vi "Get Current Position Raw.vi"(8 "error in":errorcluster, 11 "Gantry in":refnum<class "Gantry.lvclass">) -> (0 "error out":errorcluster, 2 "Vec3d Class out":refnum<class "Vec3d.lvclass">, 3 "Gantry out":refnum<class "Gantry.lvclass">)   [LabVIEW 2026, in "Gantry.lvclass"]
uses:
  Gantry.lvclass
  Vec3d Class/Vec3d.lvclass
  Gantry.lvclass/Gantry.ctl
  <instrlib>/Aerotech Automation1/Status/TypeDefs/Axis Status Items Cluster.ctl
  <instrlib>/Aerotech Automation1/Status/TypeDefs/Axis Status Item.ctl
  <instrlib>/Aerotech Automation1/Status/Wrappers/Add Axis Status Item.vi
  <instrlib>/Aerotech Automation1/Status/Wrappers/Read Axis Status Item.vi
  <instrlib>/Aerotech Automation1/Status/Status.lvlib
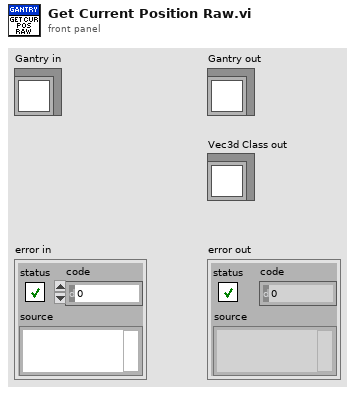
[diagram p1: front panel]
types:
  T1 = typedef "Virtual Modes.ctl" = enum16{"Nonvirtual", "Virtual"}
  T2 = typedef "ControllerDiagPacket.ctl" = cluster{"Number of Diag Packets":i32, "Axes":T3[], "error":errorcluster}
  T3 = typedef "AxisDiagPacket.ctl" = cluster{"Axis Name":string, "Analog Input 0":dbl, "Analog Input 1":dbl, "Axis Fault (num)":i32, "Axis Fault (str)":string, "Axis Fault (bits)":cluster{"AmplifierFault":bool, "AmplifierTemperatureFault":bool, "CcwEndOfTravelLimitFault":bool, "CcwSoftwareLimitFault":bool, "CommunicationLostFault":bool, "CwEndOfTravelLimitFault":bool, "CwSoftwareLimitFault":bool, "EmergencyStopFault":bool, "EncoderFault":bool, "ExternalFault":bool, "FeedbackScalingFault":bool, "GantryMisalignFault ":bool, "HallSensorFault":bool, "InPositionTimeoutFault":bool, "InternalFault":bool, "MarkerSearchFault":bool, "MaxVelocityCommandFault":bool, "MissedInterruptFault":bool, "MotorTemperatureFault":bool, "None":bool, "OverCurrentFault":bool, "PositionErrorFault":bool, "PositionFeedbackFault":bool, "PowerSupplyFault":bool, "ProbeInputFault":bool, "SafeZoneFault":bool, "VelocityErrorFault":bool, "VelocityFeedbackFault":bool, "VoltageClampFault":bool}, "Axis Status (num)":i32, "Axis Status (str)":string, "Axis Status (bits)":cluster{"BacklashActive":bool, "CalibrationEnabled1D":bool, "CalibrationEnabled2D":bool, "CommandValid":bool, "DriveAbortPending":bool, "DrivePending":bool, "Enabling":bool, "GainMappingEnabled":bool, "GantryAligned":bool, "GantryRealigning":bool, "Homed":bool, "Homing":bool, "IFOVEnabled":bool, "JogGenerating":bool, "Jogging":bool, "JoystickControl":bool, "MasterSlaveControl":bool, "MotionBlocked":bool, "MotionClamped":bool, "MoveDone":bool, "None":bool, "NotVirtual":bool, "Profiling":bool, "Stability0":bool, "Stability1":bool, "TrajectoryFiltering":bool, "WaitDone":bool}, "Current Command":sgl, "Current Error":sgl, "Current Feedback":sgl, "Digital Inputs":i32, "Digital Outputs":i32, "Drive Status":i32, "Drive Status (str)":string, "Drive Status (bits)":cluster{"AccelerationPhase":bool, "AutofocusActive":bool, "BrakeOutput":bool, "CcwEndOfTravelLimitInput":bool, "CosineEncoderError":bool, "CurrentClamp":bool, "CwEndOfTravelLimitInput":bool, "DecelerationPhase":bool, "DualLoopActive":bool, "EmergencyStopInput":bool, "Enabled":bool, "EncoderClipping":bool, "GalvoCalibrationEnabled":bool, "GalvoPowerCorrection":bool, "HallAInput":bool, "HallBInput":bool, "HallCInput":bool, "HighResolutionMode":bool, "HomeLimitInput":bool, "InPosition":bool, "InPosition2":bool, "MarkerInput":bool, "MarkerLatch":bool, "MoveActive":bool, "NoMotorSupply":bool, "None":bool, "PowerLimiting":bool, "ProgrammingFlash":bool, "ProgrammingMXH":bool, "PSOHaltLatch":bool, "ServoControl":bool, "SineEncoderError":bool}, "Position Feedback Auxiliary":dbl, "Position Command":dbl, "Position Error":dbl, "Position Feedback":dbl, "Program Position Command":dbl, "Program Position Error":dbl, "Program Position Feedback":dbl, "Velocity Command":dbl, "Velocity Error":dbl, "Velocity Feedback":dbl}
  T4 = typedef "Aerotech Automation1.lvlib/Status.lvlib/Axis Status Items Cluster.ctl" = cluster{"Axis Name":string, "axisStatusItem":T5}
  T5 = typedef "Aerotech Automation1.lvlib/Status.lvlib/Axis Status Item.ctl" = i32
  T6 = typedef "Aerotech Automation1.lvlib/Status.lvlib/Status Refnums.ctl" = cluster{"Status":refnum<k24>, "Status Config":refnum<k24>}
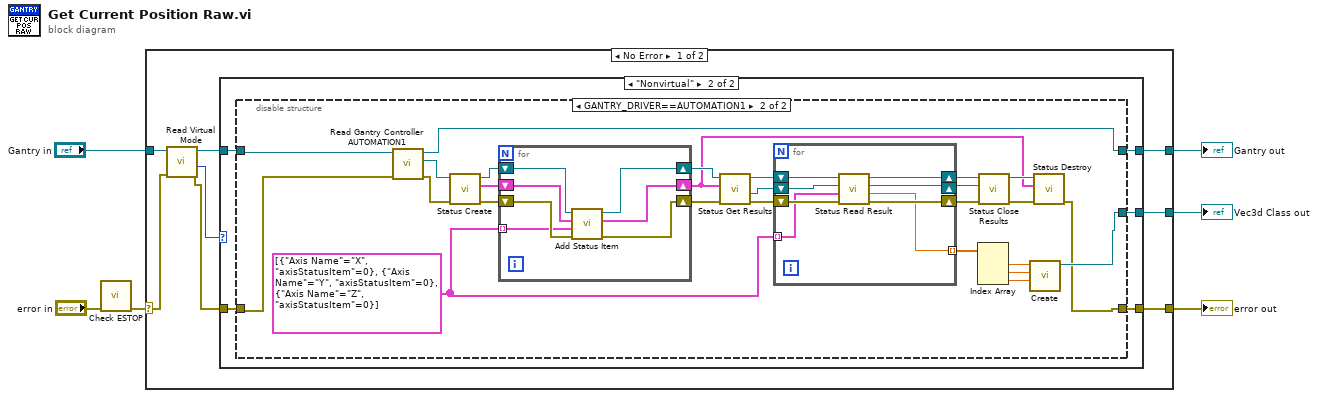
[diagram p0: block diagram]
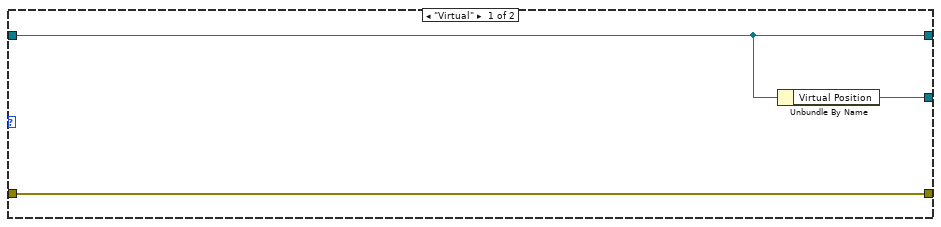
[diagram p2: hidden frame]
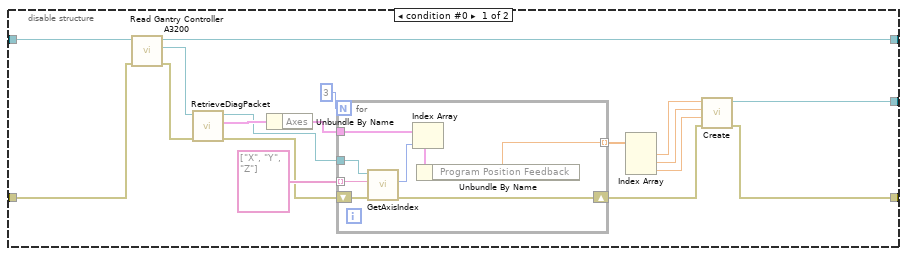
[diagram p3: hidden frame]
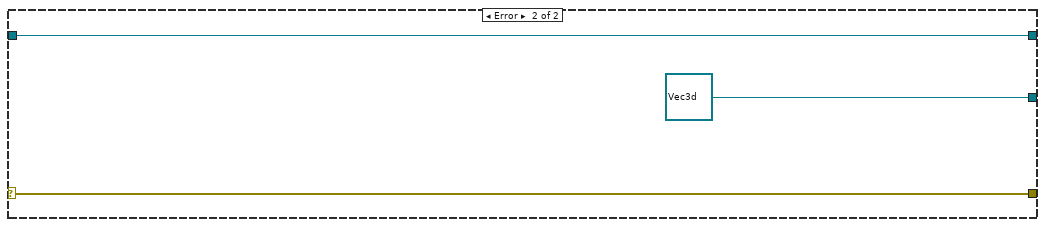
[diagram p4: hidden frame]
diagram:
  n1 = call "Check ESTOP.vi"("error in"="error in") -> ("error out"=w2:errorcluster)  [unwired: 10 in]
  n2 = case shown="No Error" w2 {
    selector: w2 -> [w9 w92]
    tunnel: [w13 w92] -> w6
    tunnel: [w12 w91] -> w5
    tunnel: "Gantry in" -> [w11 w91]
    tunnel: [w14 refnum<class "Vec3d.lvclass"> refnum ("Vec3d Class out")] -> w4
    frame No Error {
      n3 = call-dynamic "Read Virtual Mode.vi"("error in (no error)"=w9, "Gantry in"=w11) -> ("error out"=w8:errorcluster, "Virtual Mode"=w7:T1, "Gantry out"=w10:refnum<class "Gantry.lvclass">)  [unwired: 6 in, 1 out]
      n4 = case shown="\"Nonvirtual\"" w7 {
        tunnel: w8 -> [w15 w19]
        tunnel: [w16 w22] -> w14
        tunnel: [w15 w21] -> w13
        tunnel: w10 -> [w17 w20]
        tunnel: [w17 w18] -> w12
        frame "Virtual" {
          n5 = Unbundle By Name(w17) -> ("Virtual Position"=w16:refnum<class "Vec3d.lvclass">)
        }
        frame "Nonvirtual" {
          n6 = disable-structure shown="GANTRY_DRIVER==AUTOMATION1" {
            disable-tunnel: [w30 w50] -> w22
            disable-tunnel: [w28 w49] -> w21
            disable-tunnel: w20 -> [w27 w52]
            disable-tunnel: w19 -> [w26 w53]
            disable-tunnel: [w23 w51] -> w18
            frame condition #0 {
              n7 = call "Read Gantry Controller A3200.vi"("error in (no error)"=w26, "Gantry in"=w27) -> ("error out"=w25:errorcluster, "A3200 controller out"=w24:refnum<k24>, "Gantry out"=w23:refnum<class "Gantry.lvclass">)  [unwired: 7 in]
              n8 = call "RetrieveDiagPacket.vi"("error in (no error)"=w25, "Controller In"=w24) -> ("error out"=w34:errorcluster, "ControllerDiagPacket"=w40:T2, "Controller Out"=w36:refnum<k24>)  [unwired: 7 in]
              n9 = Unbundle By Name(w40) -> ("Axes"=w39:T3[])
              n10 = for {
                N: 3 -> [_]
                tunnel: w39 -> [w45]
                tunnel: [w48] -> w35 mode=indexing
                tunnel: string[] ["X", "Y", "Z"] -> [w46] mode=indexing
                shift-right: [w41] -> w29
                shift-left: w34 -> [w42]
                tunnel: w36 -> [w47]
                n11 = call "GetAxisIndex.vi"("error in (no error)"=w42, "axis name"=w46, "controller in"=w47) -> ("error out"=w41:errorcluster, "axis index"=w44:i32)  [unwired: 6 in, 1 out]
                n12 = Index Array(array=w45, index=w44) -> (element=w43:T3)
                n13 = Unbundle By Name(w43) -> ("Program Position Feedback"=w48:dbl)
              }
              n14 = Index Array(array=w35) -> (element #1=w33:dbl, element #2=w32:dbl, element #3=w31:dbl)  [unwired: 3 in]
              n15 = call "Create.vi"("error in"=w29, "Z"=w31, "Y"=w32, "X"=w33) -> ("error out"=w28:errorcluster, "Vec3d Class out"=w30:refnum<class "Vec3d.lvclass">)  [unwired: 6 in]
            }
            frame condition #1 (active) {
              w67 = T4[] [{"Axis Name"="X", "axisStatusItem"=0}, {"Axis Name"="Y", "axisStatusItem"=0}, {"Axis Name"="Z", "axisStatusItem"=0}]
              n16 = call "Read Gantry Controller AUTOMATION1.vi"("error in (no error)"=w53, "Gantry in"=w52) -> ("error out"=w73:errorcluster, "Controller AUTOMATION1"=w74:refnum<k24>, "Gantry out"=w51:refnum<class "Gantry.lvclass">)  [unwired: 7 in]
              n17 = call <instrlib>:"Status Create.vi"("error in (no error)"=w73, "Controller Refnum"=w74) -> ("error out"=w72:errorcluster, "Status Refnums"=w71:T6, "Controller Refnum out"=w70:refnum<k24>)  [unwired: 7 in]
              n18 = for {
                shift-right: [w84] -> w68
                shift-left: w72 -> [w88]
                shift-right: [w85] -> w59
                shift-left: w71 -> [w86]
                tunnel: w67 -> [w87] mode=indexing
                shift-right: [w83] -> w69
                shift-left: w70 -> [w89]
                n19 = call-poly <instrlib>:"Add Status Item.vi"("error in"=w88, "Axis Status Item"=w87, "Status Refnums"=w86, "Controller Refnum"=w89) -> ("error out"=w84:errorcluster, "Status Refnums out"=w85:T6, "Controller Refnum out"=w83:refnum<k24>)  [unwired: 5 in]
              }
              n20 = call <instrlib>:"Status Get Results.vi"("error in (no error)"=w68, "Status Refnums"=w59, "Controller Refnum"=w69) -> ("error out"=w65:errorcluster, "GetStatusItems"=w64:refnum<k24>, "Controller Refnum out"=w66:refnum<k24>)  [unwired: 5 in, 1 out]
              n21 = for {
                tunnel: w67 -> [w79] mode=indexing
                shift-right: [w78] -> w63
                shift-left: w66 -> [w82]
                shift-right: [w80] -> w60
                shift-left: w65 -> [w81]
                shift-right: [w76] -> w61
                shift-left: w64 -> [w77]
                tunnel: [w75] -> w57 mode=indexing
                n22 = call-poly <instrlib>:"Status Read Result.vi"("error in (no error)"=w81, "Axis Status Item"=w79, "Status Results Refnum"=w77, "Controller Refnum"=w82) -> ("error out"=w80:errorcluster, "Data"=w75:dbl, "Status Results Refnum out"=w76:refnum<k24>, "Controller Refnum out"=w78:refnum<k24>)  [unwired: 4 in]
              }
              n23 = Index Array(array=w57) -> (element #1=w56:dbl, element #2=w55:dbl, element #3=w54:dbl)  [unwired: 3 in]
              n24 = call <instrlib>:"Status Close Results.vi"("error in (no error)"=w60, "Status Results Refnum"=w61, "Controller Refnum"=w63) -> ("error out"=w58:errorcluster, "Controller Refnum out"=w62:refnum<k24>)  [unwired: 7 in]
              n25 = call "Create.vi"("Z"=w54, "Y"=w55, "X"=w56) -> ("Vec3d Class out"=w50:refnum<class "Vec3d.lvclass">)  [unwired: 7 in, 1 out]
              n26 = call <instrlib>:"Status Destroy.vi"("error in"=w58, "Status Refnums"=w59, "Controller Refnum"=w62) -> ("error out"=w49:errorcluster)  [unwired: 7 in, 1 out]
            }
          }
        }
      }
    }
    frame Error {
    }
  }
  "error out" <- w6
  "Gantry out" <- w5
  "Vec3d Class out" <- w4
